vi "Analysis.vi"(11 "Array in":dbl[](array[numeric])) -> ()   [LabVIEW 2011]
panel:
  out "Listbox":i32[](listbox)
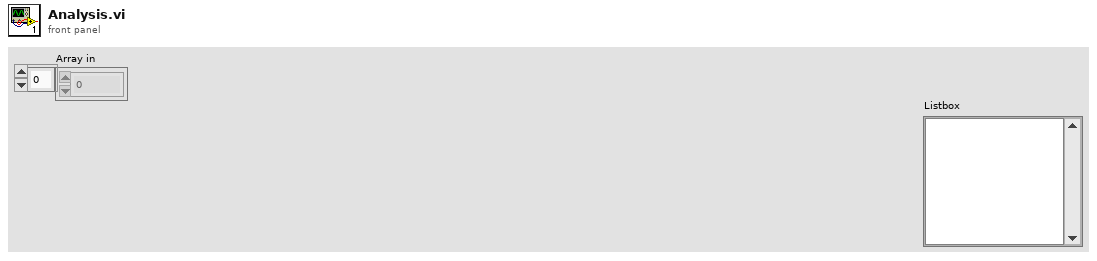
[diagram p1: front panel]
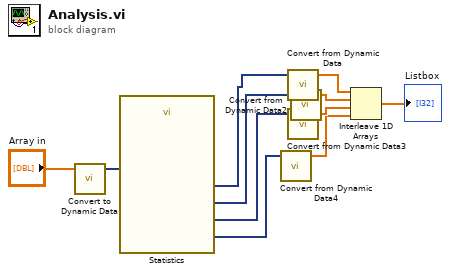
[diagram p0: block diagram]
diagram:
  n1 = call "Convert to Dynamic Data"("Array"="Array in") -> ("Dynamic Data Type"=w1:dynamicdata)  [unwired: 3 in]
  n2 = call "Statistics"("Signals"=w1) -> ("Median"=w9:dynamicdata, "Variance"=w8:dynamicdata, "Minimum"=w11:dynamicdata, "Maximum"=w10:dynamicdata)  [unwired: 22 in, 1 out]
  n3 = call "Convert from Dynamic Data4"("Dynamic Data Type"=w11) -> ("Array"=w4:dbl[])  [unwired: 3 in]
  n4 = call "Convert from Dynamic Data"("Dynamic Data Type"=w8) -> ("Array"=w7:dbl[])  [unwired: 3 in]
  n5 = call "Convert from Dynamic Data3"("Dynamic Data Type"=w10) -> ("Array"=w5:dbl[])  [unwired: 3 in]
  n6 = call "Convert from Dynamic Data2"("Dynamic Data Type"=w9) -> ("Array"=w6:dbl[])  [unwired: 3 in]
  n7 = Interleave 1D Arrays(w7, w6, w5, w4) -> (→"Listbox":dbl[])
